vi "cm_Channel Monitor Facade.vi"(0 "Data In":T6, 2 "Display State In":T3={"Chan"=[], "First Drop?"=FALSE, "Notifier Name"="", "Refresh View"=FALSE, "Scale to Input Range"=FALSE, "Linear View"=FALSE, "Display"={"Current"=6618880, "Peak"=6618880}, "Property/Method"=enum."No Update", "Time Display Ref"=[]}, 3 "Container State":T5) -> (6 "Data Out":T6, 7 "Display State Out":T3={"Chan"=[], "First Drop?"=FALSE, "Notifier Name"="", "Refresh View"=FALSE, "Scale to Input Range"=FALSE, "Linear View"=FALSE, "Display"={"Current"=6618880, "Peak"=6618880}, "Property/Method"=enum."No Update", "Time Display Ref"=[]}, 8 "Action":T2)   [LabVIEW 2012, in "Channel Monitor.xctl"]
doc: "Channel Monitor displays the peak level of multiple waveforms in a single view along with options to view the time domain data."
uses:
  Channel Monitor.xctl
  cm_Channel Monitor Data.ctl
  <vilib>/_xctls/Container State.ctl
  cm_Channel Monitor State.ctl
  TypeDef/cm_Property_Method.ctl
  <vilib>/_xctls/Action.ctl
  TypeDef/cm_Channel Indicator.ctl
  <vilib>/_xctls/XControlSupport.lvlib
panel:
  in  "Channel Status 3":T1 {"Current Level" scale=0.0..1.0; "Peak Level" scale=0.0..1.0}
  in  "Channel Status":T1[](array[typedef]) {"Current Level" scale=0.0..1.0; "Peak Level" scale=0.0..1.0}
  # "Level"
  # "Channel Name"
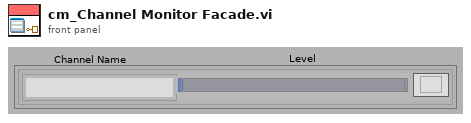
[diagram p1: front panel]
types:
  T1 = typedef "Channel Monitor.xctl/cm_Channel Indicator.ctl" = cluster{"Channel Name":string, "TimeDomain":bool, "Peak Level":dbl, "Current Level":dbl}
  T2 = typedef "XControlSupport.lvlib/Action.ctl" = cluster{"Data Changed?":bool, "State Changed?":bool, "Action Name":string}
  T3 = typedef "Channel Monitor.xctl/cm_Channel Monitor State.ctl" = cluster{"Chan":cluster{"ChanName":string, "Current":dbl, "Peak":dbl, "Input Range":dbl}[], "First Drop?":bool, "Notifier Name":string, "Refresh View":bool, "Scale to Input Range":bool, "Linear View":bool, "Display":cluster{"Current":u32, "Peak":u32}, "Property/Method":T4, "Time Display Ref":refnum<vi>[]}
  T4 = typedef "Channel Monitor.xctl/cm_Property_Method.ctl" = enum16{"No Update", "Color: Currrent", "Color: Peak", "Close Time Displays"}
  T5 = typedef "XControlSupport.lvlib/Container State.ctl" = cluster{"Indicator?":bool, "Run Mode?":bool, " Refnum":refnum<vi>}
  T6 = typedef "Channel Monitor.xctl/cm_Channel Monitor Data.ctl" = waveform(dbl)[]
  T7 = enum16{"Update All", "Current Only", "Peak Only"}
  T8 = cluster{"ChanName":string, "Current":dbl, "Peak":dbl, "Input Range":dbl}[]
  T9 = typedef "LVRectTypeDef.ctl" = cluster{"Left":i16, "Top":i16, "Right":i16, "Bottom":i16}
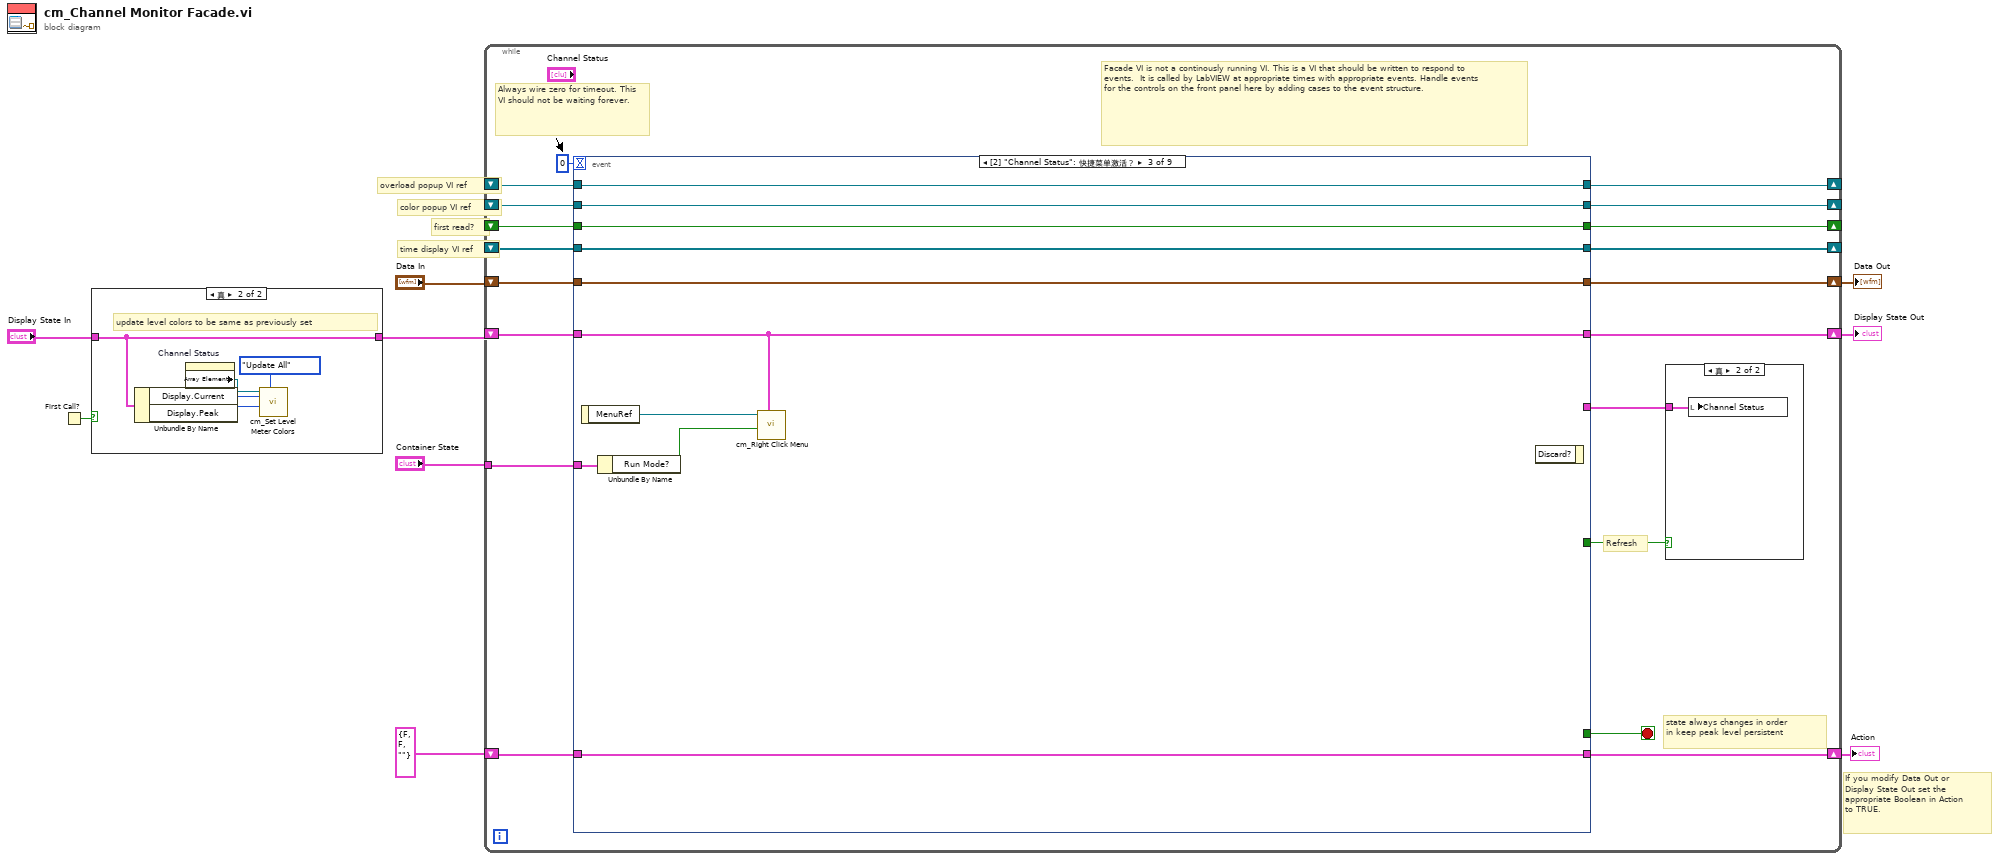
[diagram p0: block diagram]
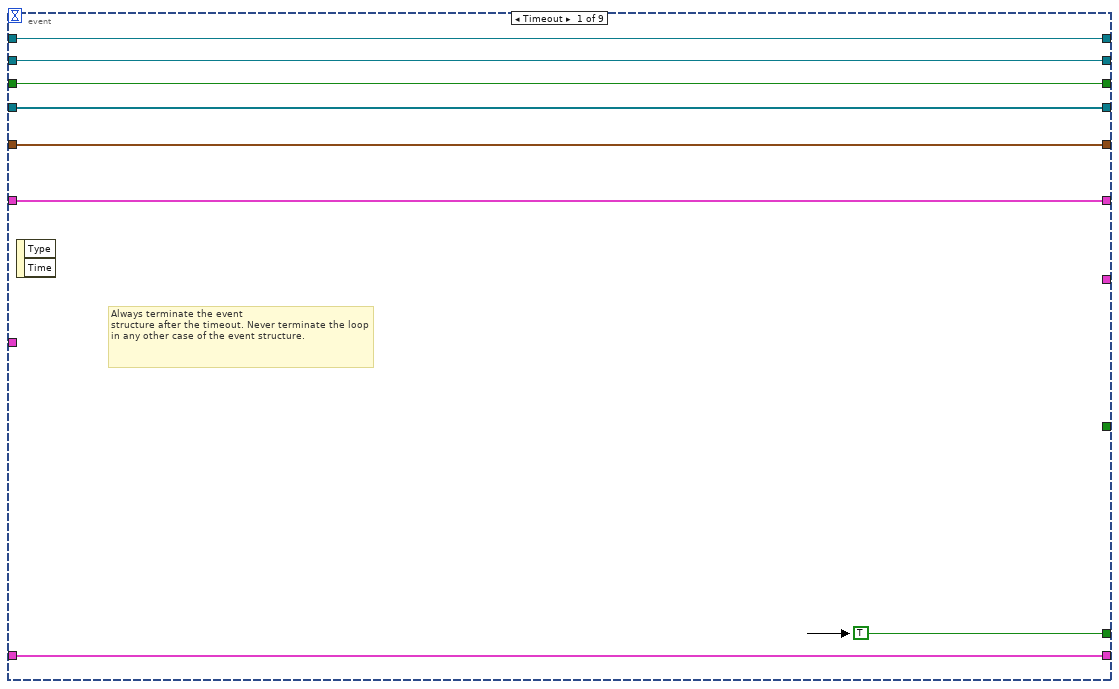
[diagram p4: hidden frame]
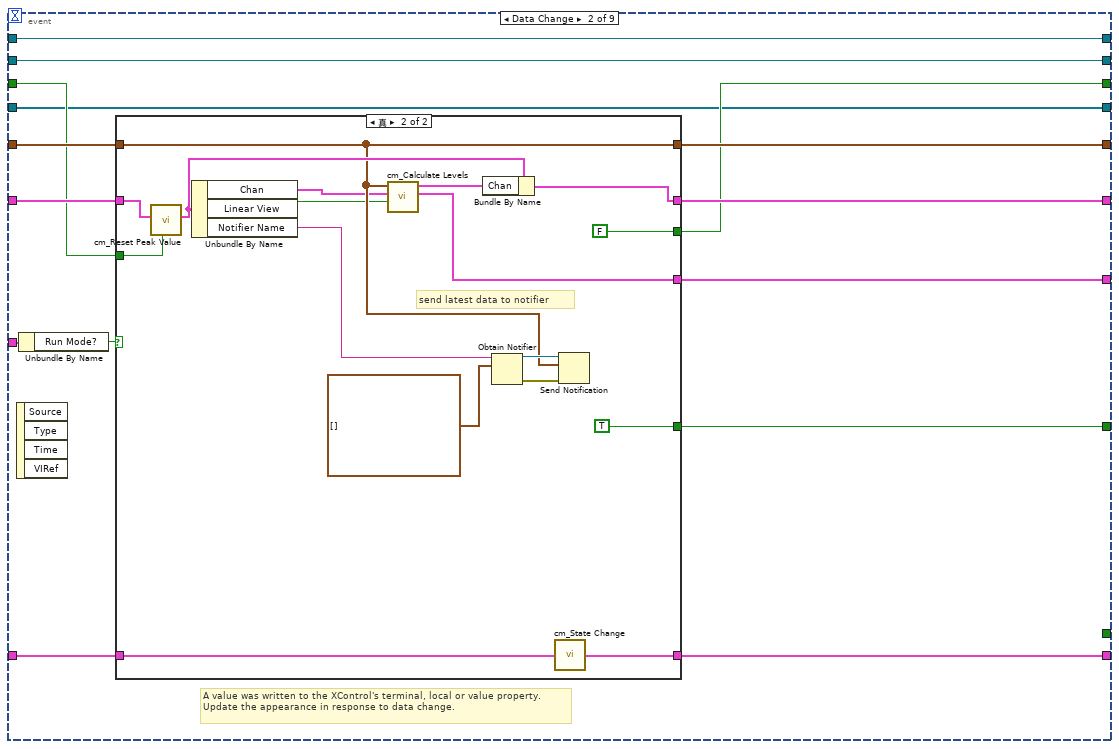
[diagram p5: hidden frame]
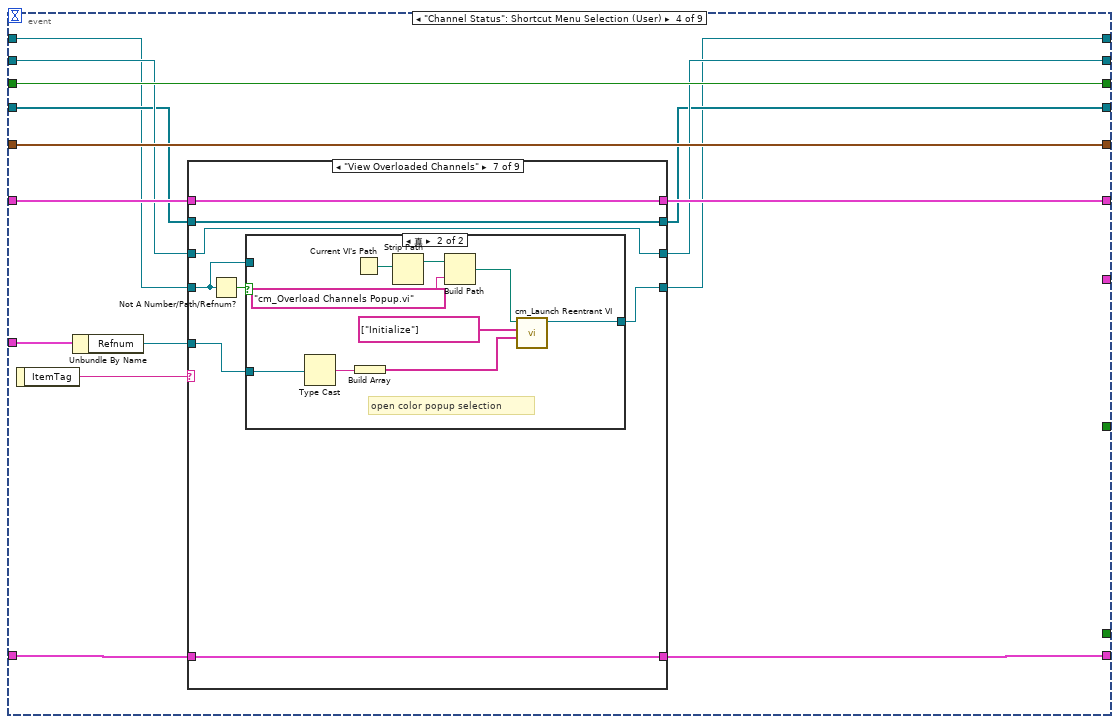
[diagram p7: hidden frame]
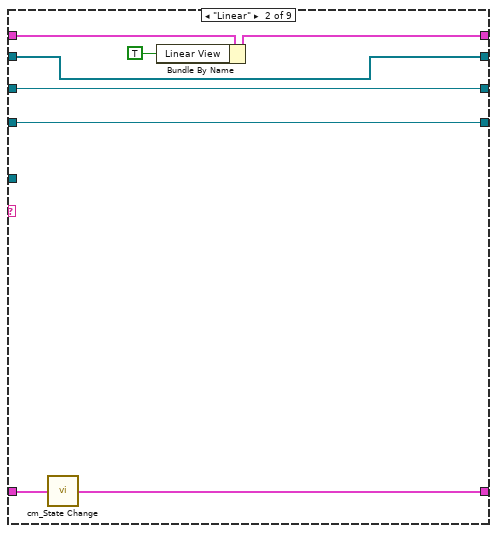
[diagram p9: hidden frame]
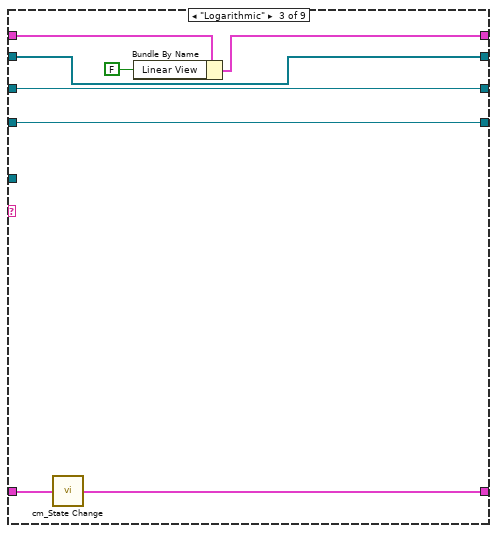
[diagram p10: hidden frame]
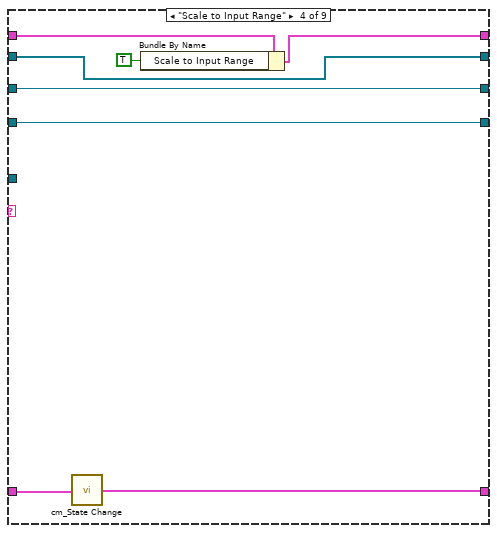
[diagram p11: hidden frame]
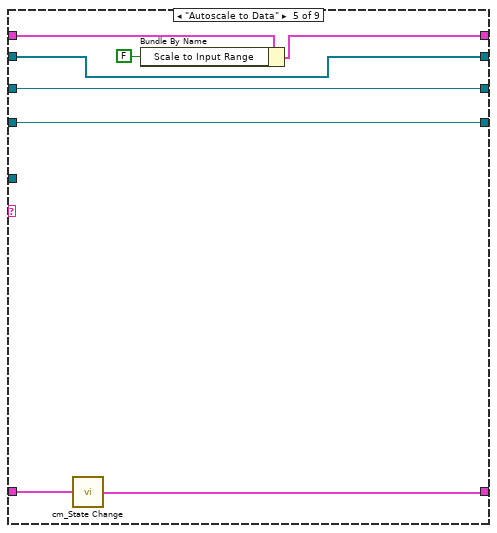
[diagram p12: hidden frame]
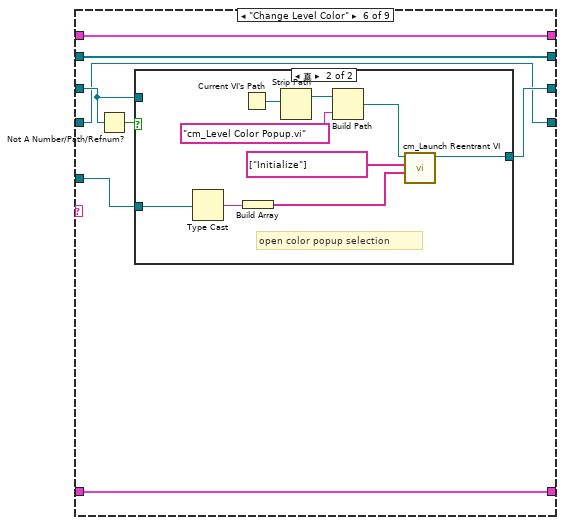
[diagram p13: hidden frame]
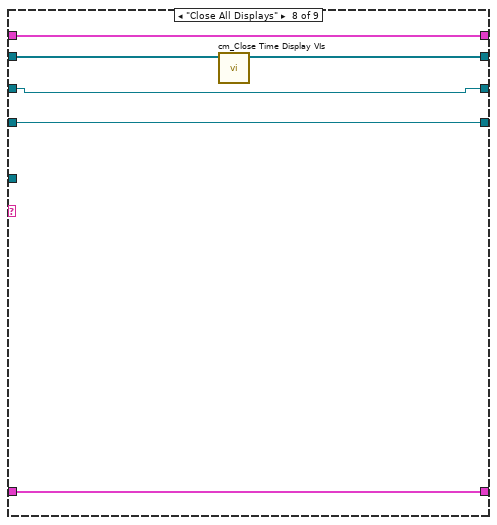
[diagram p16: hidden frame]
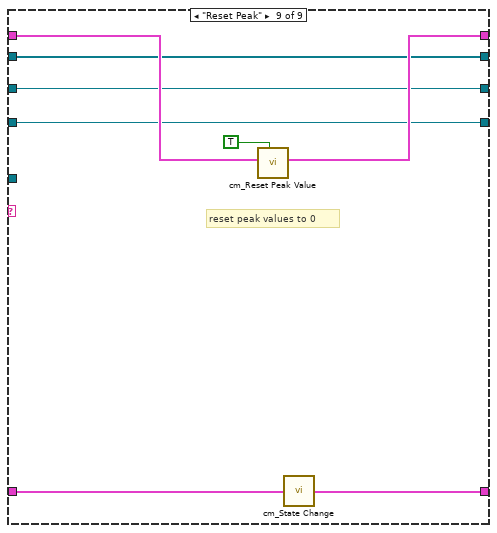
[diagram p17: hidden frame]
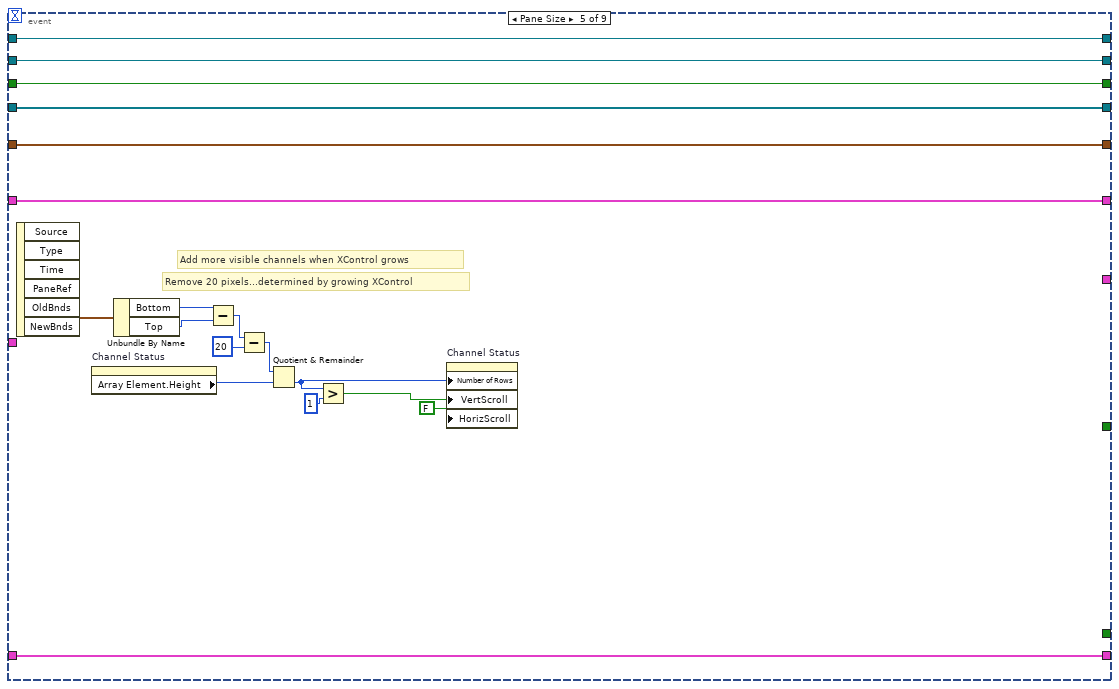
[diagram p18: hidden frame]
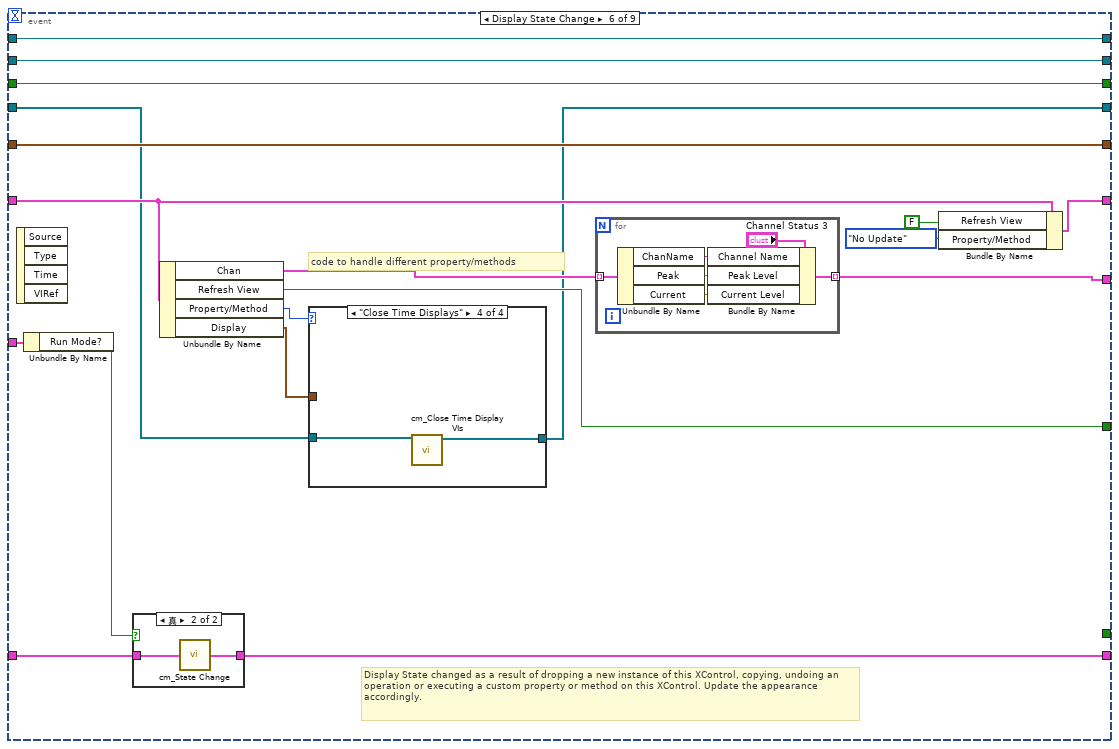
[diagram p19: hidden frame]
diagram:
  # "overload popup VI ref"
  # "color popup VI ref"
  # "first read?"
  # "time display VI ref"
  # "If you modify Data Out or\nDisplay State Out set the\nappropriate Boolean in Action\nto TRUE."
  n1 = First Call?() -> (First Call?: T/F=w3:bool)
  n2 = case shown="真" w3 {
    tunnel: "Display State In" -> [w10 w15]
    tunnel: [w10 w15] -> w1
    frame False {
    }
    frame True {
      # "update level colors to be same as previously set"
      n3 = Unbundle By Name(w15) -> ("Display.Current"=w14:u32, "Display.Peak"=w13:u32)
      n4 = property on="Channel Status" class="Arr"() -> ("Array Element"=w12:refnum<vi>)  [unwired: 2 in, 2 out]
      n5 = call "cm_Set Level Meter Colors.vi"("Action"=T7."Update All", "Peak"=w13, "Current"=w14, "Channel Status"=w12) -> ()  [unwired: 7 in, 1 out]
    }
  }
  n6 = while {
    shift-right: [w33] -> w5
    shift-left: w1 -> [w34]
    tunnel: "Container State" -> [w30]
    shift-right: [w28] -> w6
    shift-left: "Data In" -> [w29]
    shift-right: [w26] -> w4
    shift-left: T2 {"Data Changed?"=FALSE, "State Changed?"=FALSE, "Action Name"=""} ("Action") -> [w27]
    shift-right: [w23] -> _
    shift-left: _ -> [w22]
    shift-right: [w20] -> _
    shift-left: _ -> [w21]
    shift-right: [w19] -> _
    shift-left: _ -> [w18]
    shift-right: [w16] -> _
    shift-left: _ -> [w17]
    stop <- w32 stop-if-true
    # "state always changes in order\nin keep peak level persistent"
    # "Refresh"
    # "Facade VI is not a continously running VI. This is a VI that should be written to respond to events.  It is called by LabVIEW at appropriate times with appropriate events. Handle events for the controls on the front panel here by adding cases to the event structure."
    # "Always wire zero for timeout. This\nVI should not be waiting forever."
    n7 = event shown="[2] \"Channel Status\": 快捷菜单激活？" {
      selector: _ -> [_ _ _ _ _ _ _ _ _]
      dyn-events: _ -> [_ _ _ _ _ _ _ _ _]
      timeout: 0 -> [_ _ _ _ _ _ _ _ _]
      tunnel: w34 -> [w39 w58 w84 w102 w208 w218 w256 w292 w310]
      tunnel: [w39 w57 w84 w101 w208 w217 w256 w291 w310] -> w33
      tunnel: [TRUE _ _ _ _ _ _ _ _] -> w32
      tunnel: w30 -> [_ w51 w87 w97 _ w225 w258 w297 w317]
      tunnel: w29 -> [w41 w52 w89 w104 w209 w228 w266 w296 w316]
      tunnel: [w41 w49 w89 w104 w209 w228 w266 w296 w316] -> w28
      tunnel: [w42 w53 w88 w99 w207 w226 w260 w290 w314] -> w26
      tunnel: w27 -> [w42 w54 w88 w100 w207 w227 w260 w293 w314]
      tunnel: [_ w56 _ _ _ w220 TRUE _ _] -> w25
      tunnel: [_ w55 _ _ _ w221 w262 _ _] -> w24
      tunnel: [w40 w47 w86 w98 w195 w223 w257 w289 w313] -> w23
      tunnel: w22 -> [w40 w48 w86 w98 w195 w223 w257 w289 w312]
      tunnel: w21 -> [w38 w46 w85 w93 w194 w213 w254 w288 w311]
      tunnel: [w38 w46 w85 w92 w194 w212 w255 w288 w309] -> w20
      tunnel: [w37 w45 w81 w95 w193 w211 w252 w287 w308] -> w19
      tunnel: w18 -> [w37 w45 w81 w94 w193 w211 w252 w287 w308]
      tunnel: w17 -> [w36 w44 w80 w91 w192 w210 w251 w286 w307]
      tunnel: [w36 w44 w80 w90 w192 w210 w251 w286 w307] -> w16
      event Timeout {
        # "Always terminate the event\nstructure after the timeout. Never terminate the loop in any other case of the event structure."
        n8 = event-data() -> ()  [unwired: 1 in, 2 out]
      }
      event Data Change {
        # "A value was written to the XControl's terminal, local or value property.\nUpdate the appearance in response to data change."
        n9 = event-data() -> ()  [unwired: 1 in, 4 out]
        n10 = Unbundle By Name(w51) -> ("Run Mode?"=w50:bool)
        n11 = case shown="真" w50 {
          tunnel: w58 -> [w61 w74]
          tunnel: [w61 w79] -> w57
          tunnel: [_ TRUE] -> w56
          tunnel: [_ w63] -> w55
          tunnel: w54 -> [w60 w77]
          tunnel: [w60 w76] -> w53
          tunnel: w52 -> [w62 w67]
          tunnel: [w62 w67] -> w49
          tunnel: w48 -> [w59 w73]
          tunnel: [w59 FALSE] -> w47
          frame False {
          }
          frame True {
            # "send latest data to notifier"
            n12 = call "cm_Reset Peak Value.vi"("Reset Peak?"=w73, "Display State In"=w74) -> ("Display State Out"=w71:T3)  [unwired: 6 in]
            n13 = Unbundle By Name(w71) -> ("Chan"=w66:T8, "Linear View"=w65:bool, "Notifier Name"=w72:string)
            n14 = call "cm_Calculate Levels.vi"("Linear View"=w65, "Channel Info"=w66, "Data In"=w67) -> ("Channel Status"=w63:T1[], "Channel Info"=w64:T8)  [unwired: 6 in, 1 out]
            n15 = Bundle By Name(cluster=w71, "Chan"=w64) -> (w79:T3)
            n16 = Obtain Notifier(name (unnamed)=w72, notification data type=waveform(dbl)[] [] ("Waveform Graph 2")) -> (notifier out=w68:refnum<notifier>, error out=w70:errorcluster)  [unwired: 2 in, 1 out]
            n17 = call "cm_State Change.vi"("Action 2"=w77) -> ("Action"=w76:T2)  [unwired: 6 in]
            n18 = Send Notification(notification=w67, notifier=w68, error in (no error)=w70) -> ()  [unwired: 2 out]
          }
        }
      }
      event "Channel Status": Shortcut Menu Activation? {
        n19 = event-data() -> ("MenuRef"=w83:refnum<k9>)  [unwired: 1 in]
        n20 = Unbundle By Name(w87) -> ("Run Mode?"=w82:bool)
        n21 = call "cm_Right Click Menu.vi"("Display State In"=w84, "Run Mode?"=w82, "MenuRef"=w83) -> ()  [unwired: 8 in, 1 out]
        n22 = event-data() -> ()  [unwired: 2 in, 1 out]
      }
      event "Channel Status": Shortcut Menu Selection (User) {
        n23 = event-data() -> ("ItemTag"=w103:string)  [unwired: 1 in]
        n24 = Unbundle By Name(w97) -> ("Refnum"=w96:refnum<vi>)
        n25 = case shown="\"View Overloaded Channels\"" w103 {
          tunnel: w102 -> [w109 w116 w125 w133 w141 w148 w166 w182 w189]
          tunnel: [w109 w115 w124 w132 w140 w148 w166 w182 w187] -> w101
          tunnel: w100 -> [w108 w114 w122 w130 w138 w149 w167 w183 w191]
          tunnel: [w108 w113 w121 w129 w137 w149 w167 w183 w190] -> w99
          tunnel: w96 -> [_ _ _ _ _ w147 w165 _ _]
          tunnel: [w107 w112 w120 w128 w136 w146 w160 w181 w186] -> w95
          tunnel: w94 -> [w107 w112 w120 w128 w136 w144 w160 w181 w186]
          tunnel: w93 -> [w106 w111 w119 w127 w135 w143 w163 w180 w185]
          tunnel: [w106 w111 w119 w127 w135 w143 w163 w179 w185] -> w92
          tunnel: w91 -> [w105 w110 w118 w126 w134 w142 w161 w178 w184]
          tunnel: [w105 w110 w118 w126 w134 w142 w162 w178 w184] -> w90
          frame "", Default {
          }
          frame "Linear" {
            n26 = call "cm_State Change.vi"("Action 2"=w114) -> ("Action"=w113:T2)  [unwired: 6 in]
            n27 = Bundle By Name(cluster=w116, "Linear View"=TRUE) -> (w115:T3)
          }
          frame "Logarithmic" {
            n28 = call "cm_State Change.vi"("Action 2"=w122) -> ("Action"=w121:T2)  [unwired: 6 in]
            n29 = Bundle By Name(cluster=w125, "Linear View"=FALSE) -> (w124:T3)
          }
          frame "Scale to Input Range" {
            n30 = call "cm_State Change.vi"("Action 2"=w130) -> ("Action"=w129:T2)  [unwired: 6 in]
            n31 = Bundle By Name(cluster=w133, "Scale to Input Range"=TRUE) -> (w132:T3)
          }
          frame "Autoscale to Data" {
            n32 = call "cm_State Change.vi"("Action 2"=w138) -> ("Action"=w137:T2)  [unwired: 6 in]
            n33 = Bundle By Name(cluster=w141, "Scale to Input Range"=FALSE) -> (w140:T3)
          }
          frame "Change Level Color" {
            n34 = Not A Number/Path/Refnum?(number/path/refnum=w144) -> (NaN/Path/Refnum?=w145:bool)
            n35 = case shown="真" w145 {
              tunnel: w147 -> [_ w154]
              tunnel: [w150 w151] -> w146
              tunnel: w144 -> [w150 _]
              frame False {
                # "Color popup is already open...don't launch a new one."
              }
              frame True {
                # "open color popup selection"
                n36 = Type Cast(x=w154) -> (*(type *) &x=w153:string)  [unwired: 1 in]
                n37 = Current VI's Path() -> (path=w158:path)
                n38 = Build Array(w153) -> (w152:string[])
                n39 = Strip Path(path=w158) -> (stripped path=w159:path)  [unwired: 1 out]
                n40 = Build Path(base path=w159, name or relative path="cm_Level Color Popup.vi") -> (appended path=w157:path)
                n41 = call "cm_Launch Reentrant VI.vi"("Initial Message Values"=w152, "Initial Message Names"=string[] ["Initialize"], "VI path"=w157) -> ("VI Refnum"=w151:refnum<vi>)  [unwired: 7 in, 1 out]
              }
            }
          }
          frame "View Overloaded Channels" {
            n42 = Not A Number/Path/Refnum?(number/path/refnum=w161) -> (NaN/Path/Refnum?=w164:bool)
            n43 = case shown="真" w164 {
              tunnel: w165 -> [_ w172]
              tunnel: [w168 w169] -> w162
              tunnel: w161 -> [w168 _]
              frame False {
                # "Color popup is already open...don't launch a new one."
              }
              frame True {
                # "open color popup selection"
                n44 = Type Cast(x=w172) -> (*(type *) &x=w171:string)  [unwired: 1 in]
                n45 = Current VI's Path() -> (path=w176:path)
                n46 = Build Array(w171) -> (w170:string[])
                n47 = Strip Path(path=w176) -> (stripped path=w177:path)  [unwired: 1 out]
                n48 = Build Path(base path=w177, name or relative path="cm_Overload Channels Popup.vi") -> (appended path=w175:path)
                n49 = call "cm_Launch Reentrant VI.vi"("Initial Message Values"=w170, "Initial Message Names"=string[] ["Initialize"], "VI path"=w175) -> ("VI Refnum"=w169:refnum<vi>)  [unwired: 7 in, 1 out]
              }
            }
          }
          frame "Close All Displays" {
            n50 = call "cm_Close Time Display VIs.vi"("Time Display Ref in"=w180) -> ("Time Display Ref out"=w179:refnum<vi>[])  [unwired: 9 in, 1 out]
          }
          frame "Reset Peak" {
            # "reset peak values to 0"
            n51 = call "cm_Reset Peak Value.vi"("Reset Peak?"=TRUE ("First Read?"), "Display State In"=w189) -> ("Display State Out"=w187:T3)  [unwired: 6 in]
            n52 = call "cm_State Change.vi"("Action 2"=w191) -> ("Action"=w190:T2)  [unwired: 6 in]
          }
        }
      }
      event Pane Size {
        # "Remove 20 pixels...determined by growing XControl"
        # "Add more visible channels when XControl grows"
        n53 = event-data() -> ("NewBnds"=w206:T9)  [unwired: 1 in, 5 out]
        n54 = property on="Channel Status" class="Arr"() -> ("Array Element.Height"=w199:u32)  [unwired: 2 in, 2 out]
        n55 = Unbundle By Name(w206) -> ("Bottom"=w205:i16, "Top"=w204:i16)
        n56 = Subtract(x=w205, y=w204) -> (x-y=w198:i16)
        n57 = Subtract(x=w198, y=u32 20) -> (x-y=w197:u32)
        n58 = Quotient & Remainder(x=w197, y=w199) -> (floor(x/y)=w203:u32)  [unwired: 1 out]
        n59 = Greater?(x=w203, y=u32 1) -> (0:w202:bool)
        n60 = property on="Channel Status" class="Arr"("Number of Rows"=w203, "VertScroll"=w202, "HorizScroll"=FALSE ("Horizontal Scrollbar Visible")) -> ()  [unwired: 2 in, 2 out]
      }
      event Display State Change {
        # "code to handle different property/methods"
        # "Display State changed as a result of dropping a new instance of this XControl, copying, undoing an operation or executing a custom property or method on this XControl. Update the appearance accordingly."
        n61 = event-data() -> ()  [unwired: 1 in, 4 out]
        n62 = Unbundle By Name(w225) -> ("Run Mode?"=w224:bool)
        n63 = case shown="真" w224 {
          tunnel: w227 -> [w248 w250]
          tunnel: [w248 w249] -> w226
          frame False {
          }
          frame True {
            n64 = call "cm_State Change.vi"("Action 2"=w250) -> ("Action"=w249:T2)  [unwired: 6 in]
          }
        }
        n65 = Unbundle By Name(w218) -> ("Chan"=w222:T8, "Refresh View"=w220:bool, "Property/Method"=w215:T4, "Display"=w214:cluster{"Current":u32, "Peak":u32})
        n66 = case shown="\"Close Time Displays\"" w215 {
          tunnel: w214 -> [_ w234 w239 _]
          tunnel: w213 -> [w229 w230 w235 w241]
          tunnel: [w229 w230 w235 w240] -> w212
          frame "No Update", Default {
          }
          frame "Color: Currrent" {
            n67 = Unbundle By Name(w234) -> ("Current"=w232:u32)
            n68 = property on="Channel Status" class="Arr"() -> ("Array Element"=w231:refnum<vi>)  [unwired: 2 in, 2 out]
            n69 = call "cm_Set Level Meter Colors.vi"("Action"=T7."Current Only", "Current"=w232, "Channel Status"=w231) -> ()  [unwired: 8 in, 1 out]
          }
          frame "Color: Peak" {
            n70 = Unbundle By Name(w239) -> ("Peak"=w236:u32)
            n71 = property on="Channel Status" class="Arr"() -> ("Array Element"=w237:refnum<vi>)  [unwired: 2 in, 2 out]
            n72 = call "cm_Set Level Meter Colors.vi"("Action"=T7."Peak Only", "Peak"=w236, "Channel Status"=w237) -> ()  [unwired: 8 in, 1 out]
          }
          frame "Close Time Displays" {
            n73 = call "cm_Close Time Display VIs.vi"("Time Display Ref in"=w241) -> ("Time Display Ref out"=w240:refnum<vi>[])  [unwired: 9 in, 1 out]
          }
        }
        n74 = for {
          tunnel: w222 -> [w246] mode=indexing
          tunnel: [w244] -> w221 mode=indexing
          n75 = Unbundle By Name(w246) -> ("ChanName"=w245:string, "Peak"=w243:dbl, "Current"=w242:dbl)
          n76 = Bundle By Name(cluster="Channel Status 3", "Channel Name"=w245, "Peak Level"=w243, "Current Level"=w242) -> (w244:T1)
        }
        n77 = Bundle By Name(cluster=w218, "Refresh View"=FALSE, "Property/Method"=cm_Property_Method."No Update") -> (w217:T3)
      }
      event "Channel Status": Value Change {
        n78 = event-data() -> ("OldVal"=w265:T1[], "NewVal"=w264:T1[])  [unwired: 1 in, 4 out]
        n79 = Unbundle By Name(w258) -> ("Run Mode?"=w259:bool, "Refnum"=w253:refnum<vi>)
        n80 = call "cm_Channel Monitor Event Detect.vi"("New Value"=w264, "Old Value"=w265) -> ("Channel"=w263:i32, "Updated Value"=w262:T1[])  [unwired: 6 in, 2 out]
        n81 = case shown="真" w259 {
          tunnel: w263 -> [_ w281]
          tunnel: w256 -> [_ w277]
          tunnel: [w267 w275] -> w255
          tunnel: w254 -> [w267 w274]
          tunnel: w253 -> [_ w272]
          frame False {
          }
          frame True {
            # "4 bytes - channel #\n4 bytes - Xcontrol ref\n1 byte   - bool"
            # "Launch a Time Domain Display and send it some initial commands through a queue."
            n82 = Unbundle By Name(w277) -> ("Scale to Input Range"=w269:bool, "Notifier Name"=w278:string)
            n83 = Type Cast(x=w272) -> (*(type *) &x=w271:string)  [unwired: 1 in]
            n84 = Format Into String(w281) -> (resulting string=w273:string)  [unwired: 3 in, 1 out]
            n85 = Type Cast(x=w269) -> (*(type *) &x=w268:string)  [unwired: 1 in]
            n86 = Current VI's Path() -> (path=w280:path)
            n87 = Concatenate Strings(w273, w271, w268) -> (w270:string)
            n88 = Strip Path(path=w280) -> (stripped path=w279:path)  [unwired: 1 out]
            n89 = Build Path(base path=w279, name or relative path="cm_Time Domain Display.vi") -> (appended path=w282:path)
            n90 = Build Array(w270, w278) -> (w285:string[])
            n91 = call "cm_Launch Reentrant VI.vi"("Initial Message Values"=w285, "Initial Message Names"=string[] ["Initialize", "Create Notifier"], "VI path"=w282) -> ("VI Refnum"=w276:refnum<vi>)  [unwired: 7 in, 1 out]
            n92 = Build Array (concatenate)(w274, w276) -> (w275:refnum<vi>[])
          }
        }
      }
      event Direction Change {
        # "This code makes the Xcontrol always\ndrop as an indicator"
        # "The direction of the XControl changed from a control to an indicator or vice versa. Update the appearance accordingly."
        n93 = event-data() -> ()  [unwired: 1 in, 4 out]
        n94 = Unbundle By Name(w297) -> ("Refnum"=w294:refnum<vi>)
        n95 = Unbundle By Name(w292) -> ("First Drop?"=w295:bool)
        n96 = case shown="真" w295 {
          tunnel: w294 -> [_ w303]
          tunnel: w293 -> [w299 w301]
          tunnel: w292 -> [w298 w306]
          tunnel: [w298 w304] -> w291
          tunnel: [w299 w300] -> w290
          frame False {
          }
          frame True {
            n97 = Bundle By Name(cluster=w306, "First Drop?"=FALSE ("Indicator?")) -> (w304:T3)
            n98 = property class="Ctl"(reference=w303, "Indicator"=TRUE) -> ()  [unwired: 1 in, 2 out]
            n99 = call "cm_State Change.vi"("Action 2"=w301) -> ("Action"=w300:T2)  [unwired: 6 in]
          }
        }
      }
      event Exec State Change {
        # "The VI owning the XControl changed from Edit Mode  to Run Mode or vice versa.\nUpdate the appearance accordingly."
        # "Handle Edit Mode & Run Mode\ncase differently"
        n100 = event-data() -> ()  [unwired: 1 in, 4 out]
        n101 = Unbundle By Name(w317) -> ("Run Mode?"=w315:bool)
        n102 = case shown="假" w315 {
          tunnel: [w320 TRUE] -> w313
          tunnel: w312 -> [w320 _]
          tunnel: w311 -> [w318 w321]
          tunnel: [w319 w321] -> w309
          frame False {
            n103 = call "cm_Close Time Display VIs.vi"("Time Display Ref in"=w318) -> ("Time Display Ref out"=w319:refnum<vi>[])  [unwired: 9 in, 1 out]
          }
          frame True {
            # "reset the peak\nvalues"
          }
        }
      }
    }
    n104 = case shown="真" w25 {
      tunnel: w24 -> [_ w35]
      frame False {
      }
      frame True {
        n105 = local write "Channel Status"(w35) -> ()
      }
    }
  }
  "Display State Out" <- w5
  "Data Out" <- w6
  "Action" <- w4
